vi "Core Read DAQ DVR FIFO.vi"(8 "error in (no error)":errorcluster, 9 "Timeout (ms)":i32=100, 10 "Data In":refnum<data-value>[](array[refnum]), 11 "CIFTag in":refnum<class "CIF_NIChn_Fifo_DAQ.lvclass">) -> (0 "error out":errorcluster, 1 "timed out?":bool, 2 "Data Out":refnum<data-value>[](array[refnum]), 3 "CIFTag out":refnum<class "CIF_NIChn_Fifo_DAQ.lvclass">, 4 "Header":T1)   [LabVIEW 2021, in "CIF_NIChn_Fifo_DAQ.lvclass"]
uses:
  CIF_NIChn_Fifo_DAQ.lvclass
  D:/dev/CIF-LVCore/src/Channels/CIFChannels/CIFChannels.lvclass
  D:/dev/CIF-LVCore/src/Channels/CIF_NIChn/NIChn/CIF_NIChn.lvclass
  ChannelCommon/typedef/FIFO Header.ctl
  ChannelCommon/typedef/Datatype Waveform.ctl
  CIFChannels/CIFChannels.lvclass/CIFChannels.ctl
  CIFChannels/Typedef/Channel State.ctl
  CIFChannels/Typedef/Direction.ctl
  NIChn/CIF_NIChn.lvclass/CIF_NIChn.ctl
  CIF_NIChn_Fifo_DAQ.lvclass/CIF_NIChn_Fifo_DAQ.ctl
  ChannelCommon/CIFFIFO/CIFfifo.lvclass/CIFfifo.ctl
  CIFChannels/Accessors/Read Channel State.vi
  CIFChannels/Accessors/Read Direction.vi
  CIFChannels/Accessors/Write Channel State.vi
  CIFChannels/Accessors/Read Disconnect Behavior.vi
  <vilib>/CIFChannels/Top Level/Read Variable Length U8 Array.vi/81056090-23cf-424a-a716-29db01c8ef1b.vi
  <vilib>/CIFChannels/Top Level/Read Variable Length U8 Array.vi/6610cd62-0a6d-4591-8fd4-6453482a4bc1.vi
  <vilib>/CIFChannels/Top Level/Read Variable Length U8 Array.vi/93d598b0-524b-4f76-9570-a74a86ef2c6f.vi
  ChannelCommon/CIFFIFO/Accessors/Write Timeout.vi
  ChannelCommon/CIFFIFO/Flatten/DVR Unflatten.vi
  ChannelCommon/CIFFIFO/Accessors/Read Header.vi
  ChannelCommon/CIFFIFO/Accessors/Write Header.vi
  <vilib>/CIFChannels/Top Level/Read Variable Length U8 Array.vi/81056090-23cf-424a-a716-29db01c8ef1b.vi/4bc1c15b-36ab-481f-b8dd-c64075ce723a.vi
  <vilib>/CIFChannels/Top Level/Read Variable Length U8 Array.vi/81056090-23cf-424a-a716-29db01c8ef1b.vi/d83cb72b-7713-41fc-a3d1-682de79cf574.vi
  <vilib>/CIFChannels/SubVIs/Get dll Path.vi
  <vilib>/CIFChannels/Top Level/Read Variable Length U8 Array.vi/6610cd62-0a6d-4591-8fd4-6453482a4bc1.vi/c28b0ead-42ad-4072-80a2-aca7f2bd7ce3.vi
  <vilib>/CIFChannels/Top Level/Read Variable Length U8 Array.vi/93d598b0-524b-4f76-9570-a74a86ef2c6f.vi/4bc1c15b-36ab-481f-b8dd-c64075ce723a.vi
  <vilib>/CIFChannels/Top Level/Read Variable Length U8 Array.vi/93d598b0-524b-4f76-9570-a74a86ef2c6f.vi/d83cb72b-7713-41fc-a3d1-682de79cf574.vi
  ChannelCommon/Utilities/Unflatten Header.vi
  CIFCore/Common/Utilities/Add Error.vi
  <vilib>/CIF Foundation/CIF Utilities/Errors/Append Error Location.vi
  NIChn/CIF_NIChn.lvclass
  CIFChannels/CIFChannels.lvclass
  <vilib>/CIFChannels/CIFChannelCore.lvlib
  ChannelCommon/ChannelCommon.lvlib
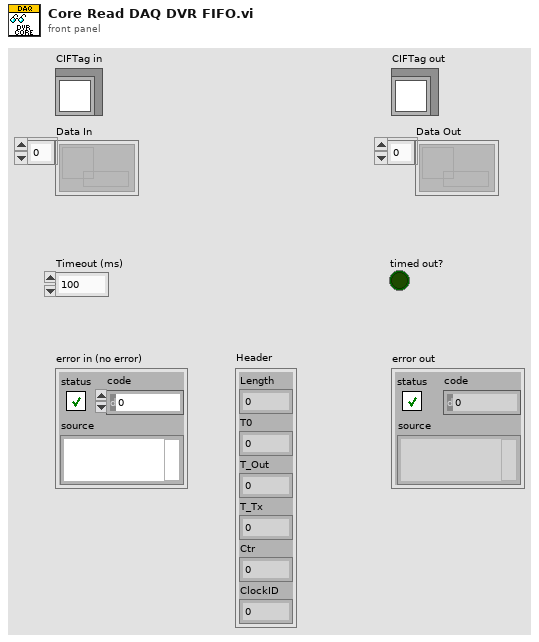
[diagram p1: front panel]
types:
  T1 = typedef "ChannelCommon.lvlib/FIFO Header.ctl" = cluster{"Length":u64, "T0":i64, "T_Out":i64, "T_Tx":i64, "Ctr":u64, "ClockID":u8}
  T2 = typedef "CIFChannels.lvclass/Channel State.ctl" = enum16{"Creating", "Disconnected", "Connecting", "Connected", "Destroyed"}
  T3 = typedef "CIFChannels.lvclass/Direction.ctl" = enum16{"Publisher", "Subscriber"}
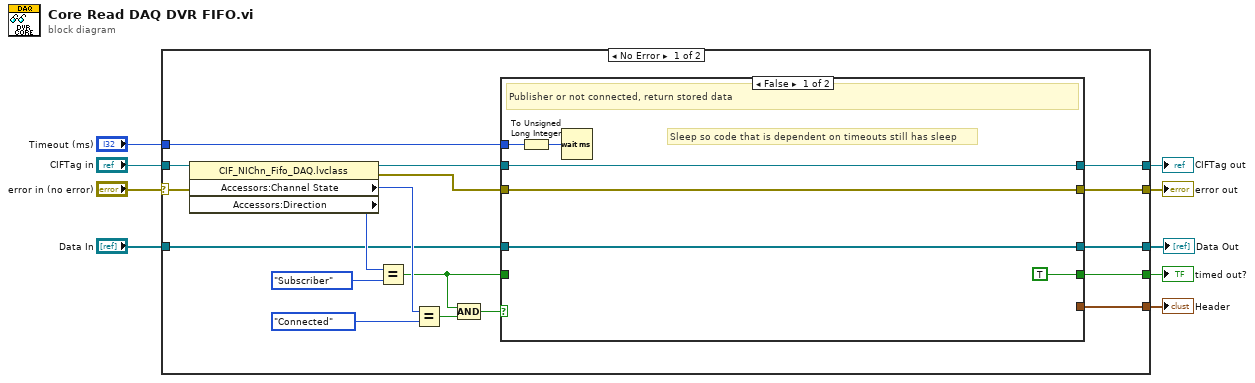
[diagram p0: block diagram]
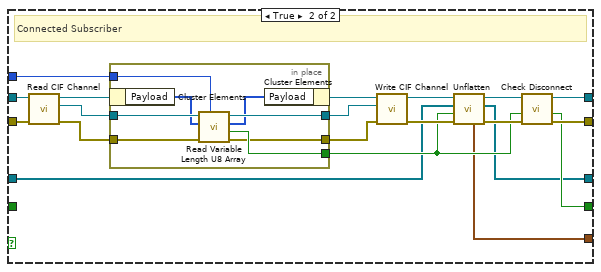
[diagram p2: hidden frame]
diagram:
  n1 = case shown="No Error" "error in (no error)" {
    selector: "error in (no error)" -> [w24 w64]
    tunnel: [w13 w64] -> w8
    tunnel: [w14 w63] -> w6
    tunnel: "CIFTag in" -> [w25 w63]
    tunnel: [w27 _] -> w5
    tunnel: [w26 w62] -> w2
    tunnel: "Timeout (ms)" -> [w12 _]
    tunnel: [w11 _] -> w3
    tunnel: "Data In" -> [w10 w62]
    frame No Error {
      n2 = property class="CIF_NIChn_Fifo_DAQ.lvclass"(reference=w25, error in=w24) -> (reference out=w23:refnum<class "CIF_NIChn_Fifo_DAQ.lvclass">, error out=w22:errorcluster, "Accessors:Channel State"=w19:T2, "Accessors:Direction"=w21:T3)
      n3 = Equal?(x=w21, y=Direction."Subscriber") -> (x = y?=w15:bool)
      n4 = Equal?(x=w19, y=Channel_State."Connected") -> (x = y?=w17:bool)
      n5 = Compound Arithmetic op=AND(w15, w17) -> (w16:bool)
      n6 = case shown="False" w16 {
        tunnel: [TRUE ("timeout out") w43] -> w27
        tunnel: [w30 w36] -> w26
        tunnel: w22 -> [w32 w52]
        tunnel: w23 -> [w33 w53]
        tunnel: w15 -> [_ _]
        tunnel: [w33 w51] -> w14
        tunnel: [w32 w50] -> w13
        tunnel: w12 -> [w29 w42]
        tunnel: [_ w35] -> w11
        tunnel: w10 -> [w30 w34]
        frame False {
          # "Sleep so code that is dependent on timeouts still has sleep"
          # "Publisher or not connected, return stored data"
          n7 = To Unsigned Long Integer(number=w29) -> (unsigned 32bit integer=w28:u32)
          n8 = Wait (ms)(milliseconds to wait=w28) -> ()  [unwired: 1 out]
        }
        frame True {
          # "Connected Subscriber"
          n9 = call "Read CIF Channel.vi"("error in (no error)"=w52, "CIFTag in"=w53) -> ("error out"=w47:errorcluster, "CIF Channel"=w48:refnum<k21>, "CIFTag out"=w49:refnum<class "CIF_NIChn_Fifo_DAQ.lvclass">)  [unwired: 7 in]
          n10 = in-place {
            in-place-border: [w59] -> w37
            in-place-border: w48 -> [w61]
            in-place-border: w47 -> [w60]
            in-place-border: [w58] -> w44
            in-place-border: [w57] -> w45
            in-place-border: w42 -> [w56]
            n11 = in-place-cluster #1(w49) -> ("Payload"=w55:u8[])
            n12 = call <vilib>:"Read Variable Length U8 Array.vi"("Timeout (ms)"=w56, "error in"=w60, "Payload in"=w55, "CIF Channel in"=w61) -> ("error out"=w57:errorcluster, "Timed out?"=w59:bool, "Payload out"=w54:u8[], "CIF Channel out"=w58:refnum<k21>)  [unwired: 4 in]
            n13 = in-place-cluster #1("Payload"=w54) -> (w46:refnum<class "CIF_NIChn_Fifo_DAQ.lvclass">)
          }
          n14 = call "Write CIF Channel.vi"("error in (no error)"=w45, "CIF Channel"=w44, "CIFTag in"=w46) -> ("error out"=w40:errorcluster, "CIFTag out"=w41:refnum<class "CIF_NIChn_Fifo_DAQ.lvclass">)  [unwired: 7 in]
          n15 = call "Unflatten.vi"("error in (no error)"=w40, "timeout in"=w37, "Data In"=w34, "CIFFifoCAN in"=w41) -> ("error out"=w38:errorcluster, "Data Out"=w36:refnum<data-value>[], "CIFFifoCAN out"=w39:refnum<class "CIF_NIChn_Fifo_DAQ.lvclass">, "Header"=w35:T1)  [unwired: 4 in]
          n16 = call "Check Disconnect.vi"("error in (no error)"=w38, "timeout in"=w37, "CIFTag in"=w39) -> ("error out"=w50:errorcluster, "timeout out"=w43:bool, "CIFTag out"=w51:refnum<class "CIF_NIChn_Fifo_DAQ.lvclass">)  [unwired: 5 in, 1 out]
        }
      }
    }
    frame Error {
    }
  }
  "error out" <- w8
  "CIFTag out" <- w6
  "timed out?" <- w5
  "Header" <- w3
  "Data Out" <- w2
